vi "Do.vi"(8 "error in (no error)":errorcluster, 10 "Actor in":refnum<class "Actor.lvclass">, 11 "Leak Actor State Msg":refnum<class "Leak Viewable State Msg.lvclass">) -> (0 "error out":errorcluster, 2 "Actor out":refnum<class "Actor.lvclass">)   [LabVIEW 2017, in "ViewableDoubles.lvlib" / "Leak Viewable State Msg.lvclass"]
doc: "This VI delivers the message to the actor by calling the appropriate method(s) on the actor."
uses:
  Leak Viewable State Msg.lvclass
  <vilib>/ActorFramework/Actor/Actor.lvclass
  LeakyViewable/LeakyViewable.lvclass
  C:/Program Files (x86)/National Instruments/LabVIEW 2017/vi.lib/ActorFramework/Actor/Actor.lvclass
  LeakyViewable/Leak Location.ctl
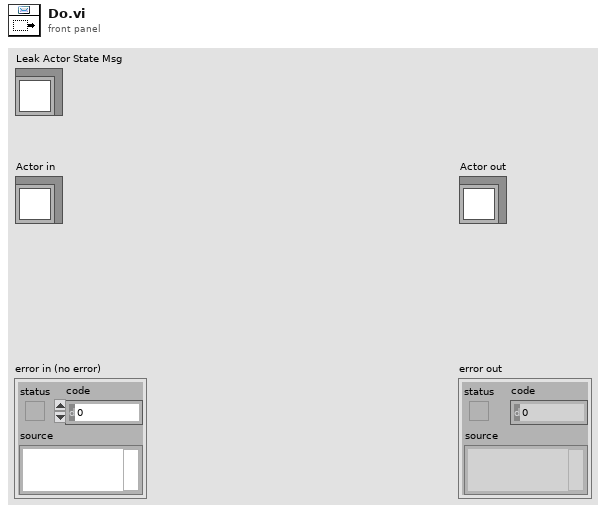
[diagram p1: front panel]
types:
  T1 = typedef "ViewableDoubles.lvlib/LeakyViewable.lvclass/Leak Location.ctl" = enum16{"Pre Launch Init", "Entering Actor Core", "Actor Core", "Exiting Actor Core", "Stop Core", "Handle Error"}
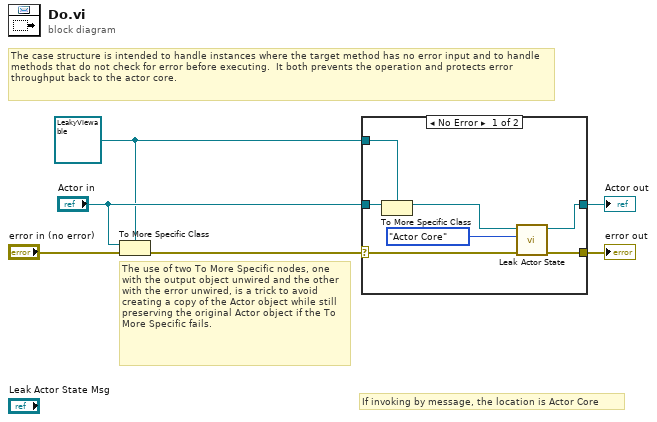
[diagram p0: block diagram]
diagram:
  w1 = refnum<class "LeakyViewable.lvclass"> refnum ("Actor in")
  # "If invoking by message, the location is Actor Core"
  # "The use of two To More Specific nodes, one with the output object unwired and the other with the error unwired, is a trick to avoid creating a copy of the Actor object while still preserving the original Actor object if the To More Specific fails."
  # "The case structure is intended to handle instances where the target method has no error input and to handle methods that do not check for error before executing.  It both prevents the operation and protects error throughput back to the actor core."
  n1 = To More Specific Class(target class=w1, reference="Actor in", error in="error in (no error)") -> (error out=w5:errorcluster)  [unwired: 1 out]
  n2 = case shown="No Error" w5 {
    selector: w5 -> [w11 w15]
    tunnel: [w13 w15] -> w4
    tunnel: [w12 w14] -> w3
    tunnel: "Actor in" -> [w10 w14]
    tunnel: w1 -> [w9 _]
    frame No Error {
      n3 = To More Specific Class(target class=w9, reference=w10) -> (specific class reference=w8:refnum<class "LeakyViewable.lvclass">)  [unwired: 1 in, 1 out]
      n4 = call "Leak Actor State.vi"("error in (no error)"=w11, "Location"=Leak_Location."Actor Core", "ViewableOne in"=w8) -> ("error out"=w13:errorcluster, "ViewableOne out"=w12:refnum<class "LeakyViewable.lvclass">)  [unwired: 7 in]
    }
    frame Error {
      # "If type check fails, pass the original object out again."
    }
  }
  "error out" <- w4
  "Actor out" <- w3
